vi "FTW-CodeGen-GetTypeInfo.vi"(0 "XRef":refnum<vi>, 5 "Type Information In":variant, 11 "error in":errorcluster) -> (6 "Safe Type Information for this Context":variant, 8 "Data Name":string, 10 "Data Type Color":u32(colorbox), 15 "error out":errorcluster)   [LabVIEW 2014]
panel:
  # "Inputs"
  # "Outputs"
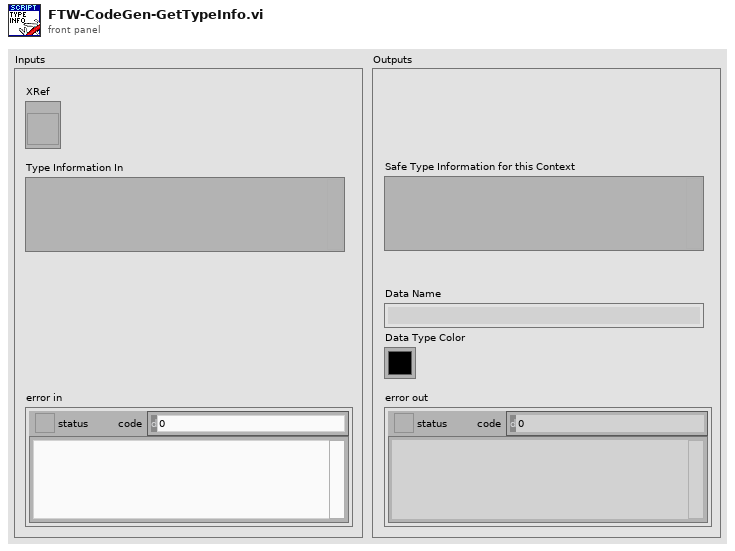
[diagram p1: front panel]
types:
  T1 = typedef "FTW-Reflection-Types.ctl" = enum16{"Unknown", "Void", "Array", "Cluster", "LVObject", "Boolean", "I8", "I16", "I32", "I64", "U8", "U16", "U32", "U64", "SGL", "DBL", "EXT", "CSG", "CDB", "CXT", "FXP", "EnumU8", "EnumU16", "EnumU32", "EnumU64", "SGLwithUnit", "DBLwithUnit", "EXTwithUnit", "CSGwithUnit", "CDBwithUnit", "CXTwithUnit", "String", "Path", "Picture", "Tag", "LVVariant", "Timestamp", "WaveformI8", "WaveformI16", "WaveformI32", "WaveformI64", "WaveformU8", "WaveformU16", "WaveformU32", "WaveformU64", "WaveformSGL", "WaveformDBL", "WaveformEXT", "WaveformCSG", "WaveformCDB", "WaveformCXT", "WaveformDigital", "WaveformUnknownType", "DigitalData", "DynamicData", "ExternalData", "FileByteStream", "TDMStream", "dotNET", "ActiveX", "VIServerReference", "VIReference", "ApplicationInstance", "Menu", "ConnectionDataSocket", "ConnectionVISA", "ConnectionBluetooth", "ConnectionIrDA", "ConnectionTCP", "ConnectionUDP", "ConnectionHTTPClient", "ConnectionFTP", "Occurrence", "Notifier", "Queue", "Rendezvous", "Semaphore", "RTFIFO", "EventPublisher", "EventRegistration", "EventCallback", "DataValueReference", "GenericClass", "GenericClassTag", "GenericClassDeepCopy", "GenericClassFlattened", "GenericClassTagFlattened", "GenericReferenceType", "WindowsRegistry", "OverloadedDatalogRef", "ReferenceUnknownType"}
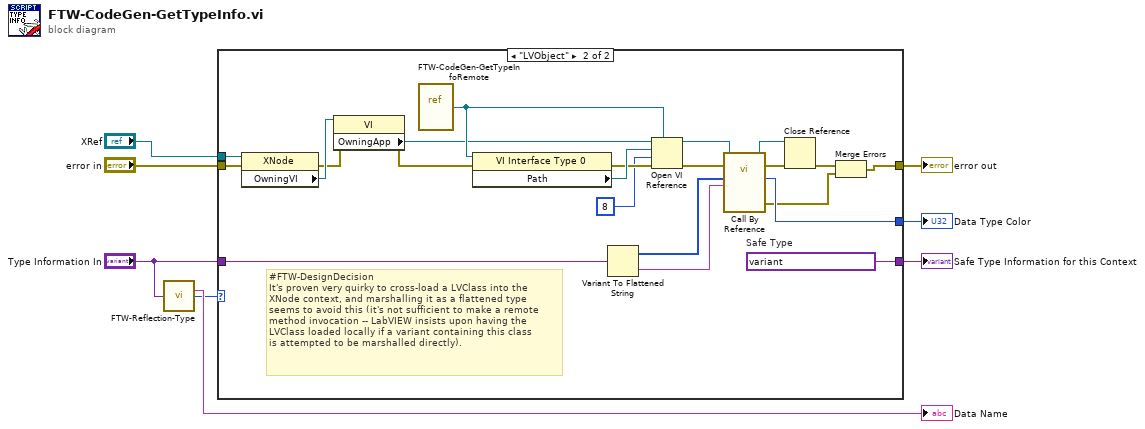
[diagram p0: block diagram]
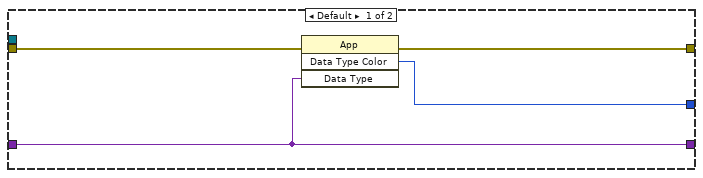
[diagram p2: hidden frame]
diagram:
  n1 = call "FTW-Reflection-Type.vi"("Anything"="Type Information In") -> ("Data Name"=→"Data Name":string, "LabVIEW Type"=w1:T1)  [unwired: 12 in, 1 out]
  n2 = case shown="\"LVObject\"" w1 {
    tunnel: "XRef" -> [_ w31]
    tunnel: "Type Information In" -> [w9 w26]
    tunnel: [w9 w23] -> w5
    tunnel: [w11 w22] -> w4
    tunnel: [w10 w20] -> w3
    tunnel: "error in" -> [w12 w19]
    frame Default {
      n3 = invoke class="App" method="Data Type Color"(error in=w12, "Data Type"=w9) -> (error out=w10:errorcluster, "Data Type Color"=w11:u32)  [unwired: 2 in, 2 out]
    }
    frame "LVObject" {
      w23 = variant(refnum<class> refnum)  # Safe Type
      # "#FTW-DesignDecision\nIt's proven very quirky to cross-load a LVClass into the\nXNode context, and marshalling it as a flattened type\nseems to avoid this (it's not sufficient to make a remote\nmethod invocation -- LabVIEW insists upon having the\nLVClass loaded locally if a variant containing this class\nis attempted to be marshalled directly)."
      n4 = property class="XNode"(reference=w31, error in=w19) -> (error out=w30:errorcluster, "OwningVI"=w34:refnum<vi>)  [unwired: 1 out]
      n5 = property class="VI"(reference=w34, error in=w30) -> (error out=w28:errorcluster, "OwningApp"=w24:refnum<vi>)  [unwired: 1 out]
      n6 = vi-ref "FTW-CodeGen-GetTypeInfoRemote.vi"() -> (w33:refnum<vi>)
      n7 = property class="VI Interface Type 0"(reference=w33, error in=w28) -> (error out=w29:errorcluster, "Path"=w32:path)  [unwired: 1 out]
      n8 = Variant To Flattened String(Variant=w26) -> (data string=w17:string, 1:w18:i16[])
      n9 = Open VI Reference(type specifier VI Refnum (for type only)=w33, application reference (local)=w24, vi path=w32, options=8, error in (no error)=w29) -> (vi reference=w25:refnum<vi>, error out=w27:errorcluster)  [unwired: 1 in]
      n10 = call-by-ref "?"(reference=w25, error in=w27, "Type Descriptor"=w18, "Type Data"=w17) -> (reference out=w15:refnum<vi>, error out=w14:errorcluster, "Data Type Color"=w22:u32, 15:"error out"=w16:errorcluster)  [unwired: 12 in]
      n11 = Close Reference(reference=w15, error in (no error)=w14) -> (error out=w13:errorcluster)
      n12 = Merge Errors(w13, w16) -> (w20:errorcluster)
    }
  }
  "Data Type Color" <- w4
  "Safe Type Information for this Context" <- w5
  "error out" <- w3
